vi "Information.vi"(8 "error in (no error)":errorcluster, 9 "Context":T1, 10 "Information":refnum<class "Information.lvclass">, 11 "Stepper in":refnum<class "Stepper.lvclass">) -> (0 "error out":errorcluster, 3 "Stepper out":refnum<class "Stepper.lvclass">)   [LabVIEW 2021, in "Stepper.lvclass"]
uses:
  Stepper.lvclass
  Publish-Subscribe/Interfaces/Information/Information.lvclass
  Publish-Subscribe/Context.ctl
  NHMFL_Core/Libraries/Instruments/Results/Acquired Result/Acquired Result.lvclass
  NHMFL_Core/Libraries/Instruments/Results/Acquired Result/Acquired Result.lvclass/Acquired Result.ctl
  NHMFL_Core/Libraries/Instruments/Results/Acquired Result/Write Group.vi
  Measurements/Response Synchronizer/Response Synchronizer.lvclass
  NHMFL_Core/Libraries/Instruments/Results/Combined Result/Combined Result.lvclass
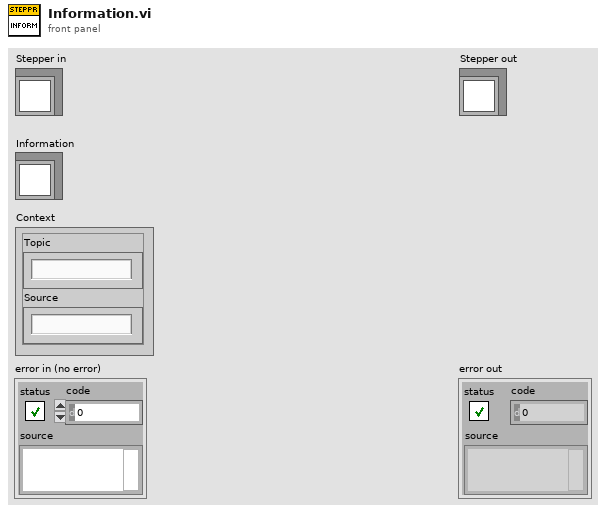
[diagram p1: front panel]
types:
  T1 = typedef "Context.ctl" = cluster{"Topic":string, "Source":string}
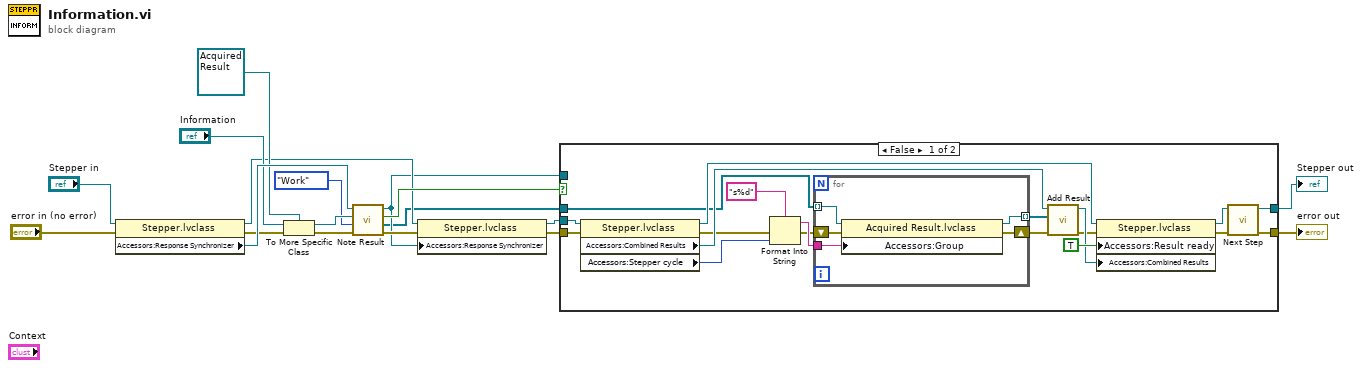
[diagram p0: block diagram]
diagram:
  n1 = property class="Stepper.lvclass"(reference="Stepper in", error in="error in (no error)") -> (reference out=w5:refnum<class "Stepper.lvclass">, error out=w12:errorcluster, "Accessors:Response Synchronizer"=w17:refnum<class "Response Synchronizer.lvclass">)
  n2 = To More Specific Class(target class=refnum<class "Acquired Result.lvclass"> refnum ("Acquired Result.lvclass"), reference="Information", error in=w12) -> (specific class reference=w16:refnum<class "Acquired Result.lvclass">, error out=w11:errorcluster)
  n3 = call-dynamic "Note Result.vi"("error in (no error)"=w11, "Stage"=enum16{"Init", "Work"}."Work", "Acquired Result.lvclass"=w16, "Response Synchronizer in"=w17) -> ("error out"=w8:errorcluster, "Results"=w1:refnum<class "Acquired Result.lvclass">[], "Awaiting results"=w9:bool, "Response Synchronizer out"=w2:refnum<class "Response Synchronizer.lvclass">)  [unwired: 4 in]
  n4 = property class="Stepper.lvclass"(reference=w5, error in=w8, "Accessors:Response Synchronizer"=w2) -> (reference out=w4:refnum<class "Stepper.lvclass">, error out=w6:errorcluster)
  n5 = case shown="False" w9 {
    tunnel: w6 -> [w36 w44]
    tunnel: [w37 w44] -> w3
    tunnel: w4 -> [w31 w43]
    tunnel: [w35 w43] -> w7
    tunnel: w2 -> [_ _]
    tunnel: w1 -> [w27 _]
    frame False {
      n6 = property class="Stepper.lvclass"(reference=w31, error in=w36) -> (reference out=w30:refnum<class "Stepper.lvclass">, error out=w23:errorcluster, "Accessors:Combined Results"=w29:refnum<class "Combined Result.lvclass">, "Accessors:Stepper cycle"=w24:i32)
      n7 = Format Into String(format string="s%d", error in=w23, w24) -> (resulting string=w25:string, error out=w22:errorcluster)  [unwired: 1 in]
      n8 = for {
        tunnel: w27 -> [w40] mode=indexing
        tunnel: w25 -> [w42]
        tunnel: [w39] -> w21 mode=indexing
        shift-right: [w38] -> w20
        shift-left: w22 -> [w41]
        n9 = property class="Acquired Result.lvclass"(reference=w40, error in=w41, "Accessors:Group"=w42) -> (reference out=w39:refnum<class "Acquired Result.lvclass">, error out=w38:errorcluster)
      }
      n10 = call-dynamic "Add Result.vi"("error in (no error)"=w20, "Results to add"=w21, "Combined Result in"=w29) -> ("error out"=w19:errorcluster, "Combined Result out"=w28:refnum<class "Combined Result.lvclass">)  [unwired: 7 in]
      n11 = property class="Stepper.lvclass"(reference=w30, error in=w19, "Accessors:Result ready"=TRUE ("Result ready"), "Accessors:Combined Results"=w28) -> (reference out=w33:refnum<class "Stepper.lvclass">, error out=w34:errorcluster)
      n12 = call-dynamic "Next Step.vi"("error in (no error)"=w34, "Stepper in"=w33) -> ("error out"=w37:errorcluster, "Stepper out"=w35:refnum<class "Stepper.lvclass">)  [unwired: 8 in]
    }
    frame True {
    }
  }
  "error out" <- w3
  "Stepper out" <- w7
